vi "temp.vi"() -> ()   [LabVIEW 2013]
panel:
  out "XY Graph":cluster{"X":dbl, "Y":dbl}[](graph)
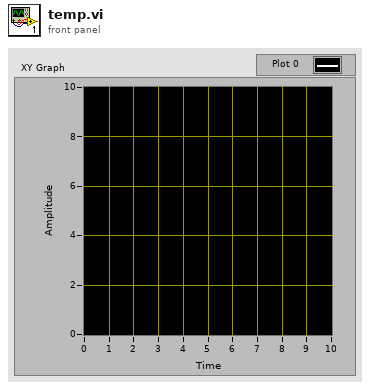
[diagram p1: front panel]
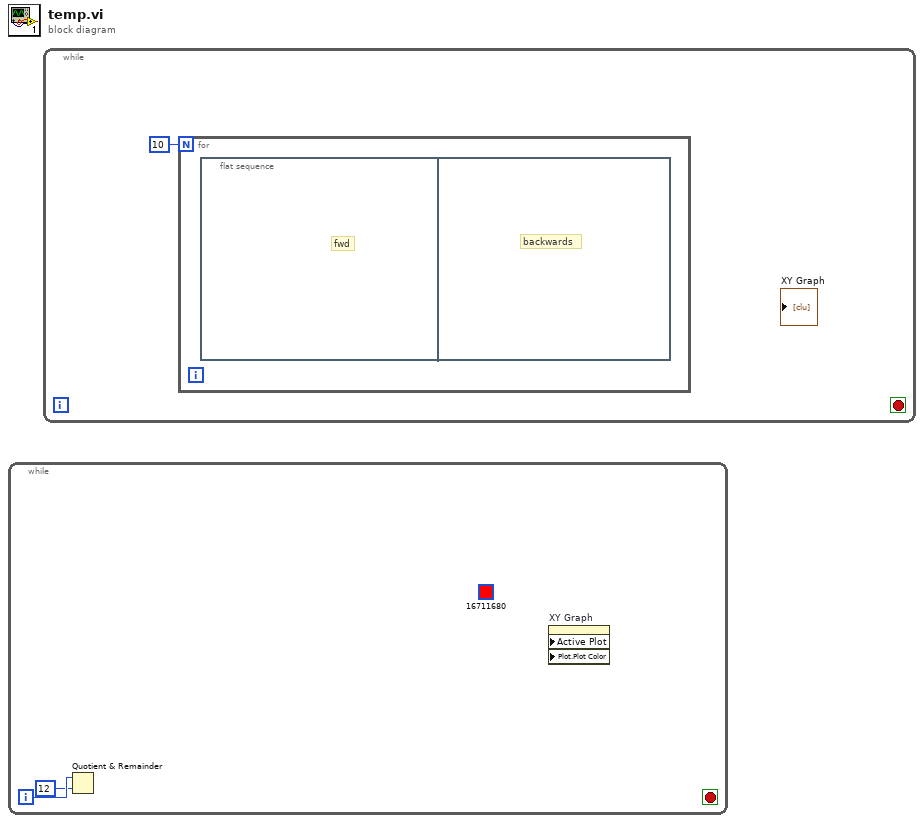
[diagram p0: block diagram]
diagram:
  n1 = while {
    i -> [w2]
    stop <- _ stop-if-true
    (unwired) u32 16711680
    n2 = Quotient & Remainder(x=w2, y=12) -> ()  [unwired: 2 out]
    n3 = property on="XY Graph" class="XYGraph (strict)" props=["Active Plot", "Plot", "Plot Color"]() -> ()  [unwired: 4 in, 2 out]
  }
  n4 = while {
    stop <- _ stop-if-true
    n5 = for {
      N: 10 -> [_]
      n6 = flat-sequence {
        frame #0 {
          # "fwd"
        }
        frame #1 {
          # "backwards"
        }
      }
    }
  }
